vi "CRYStatistics Curve Op.vi"(0 "Data in":T1={"Name"="", "Curve"=[], "X data"=1, "Y data"=1, "Z data"=1, "X axis"=0, "Y axis"=1, "Z axis"=1, "X unit"="Hz", "Y unit"="", "Z unit"="deg.", "X dB ref"=1.0, "Y dB ref"=1.0, "Z dB ref"=1.0, "single val"=FALSE, "protected"=FALSE, "display X"=TRUE, "display Y"=TRUE, "display Z"=TRUE, "Test Info"="", "Step No."=0, "Plot Settings"={"Color"=0, "Interpolation"=0, "Point Style"=0, "Line Style"=0, "Point Color"=0, "Line Width"=0, "Bar Plot Style"=0, "Fill To"=0}, "AutoProtect"=FALSE} {"Z data" items=["dB", "Lin"]; "X data" items=["dB", "Lin"]; "Y data" items=["dB", "Lin"]; "Z dB ref" format="%.1f"; "Z axis" items=["Log", "Lin"]; "X dB ref" format="%.1f"; "X axis" items=["Log", "Lin"]; "Y axis" items=["Log", "Lin"]; "Y dB ref" format="%.1f"; "Curve"."z" format="%.2f"; "Curve"."y" format="%.2f"; "Curve"."x" format="%.2f"}, 1 "Sampling Rate":dbl, 2 "work in statics":u16, 4 "Statistical Operator":u16(ring) items=["Average", "Power Sum", "Maximum", "Minimum", "Est. Resonance", "Est. Notch", "IEEE TOLP", "IEEE ROLP", "IEEE SOLP", "ITU-T SLR", "ITU-T RLR", "ITU-T RLR w/Leak", "ITU-T STMR", "Attack Time", "Release Time", "Zwicker Loudness"], 5 "Wave":T4={"Waveform"={"X0"=0.0, "dX"=0.0, "Y"=[]}, "X data"=1, "Y data"=1, "Y axis"=1, "X unit"="s", "Y unit"="V", "Y dB ref"=1.0, "display Y"=TRUE, "display X"=TRUE, "Overload?"=FALSE, "Test Info"="", "Step No."=0, "Name"="", "protected"=FALSE, "Sqc history"=[], "Signal Channel ID"=0, "Plot Settings"={"Color"=0, "Interpolation"=0, "Point Style"=0, "Line Style"=0, "Point Color"=0, "Line Width"=0, "Bar Plot Style"=0, "Fill To"=0}, "AutoProtect"=FALSE} {"Y dB ref" format="%.1f"; "Y axis" items=["Log", "Lin"]; "Y data" items=["dB", "Lin"]; "X data" items=["dB", "Lin"]}, 7 "Search range":string[](array[string]), 8 "weight curve":string, 9 "All points":bool, 10 "Zwicker_spectrum":bool, 11 "Zwicker_X-axis":u16(ring) items=["Hz", "Bark"], 12 "Para_Resonance(%)":sgl format="%.2f", 13 "Use Default Value":bool, 14 "Curve/WFM ?":bool, 15 "Exponent":dbl) -> (17 "Q":dbl format="%.2f", 19 "Ranged data out(Curve)":T1={"Name"="", "Curve"=[], "X data"=1, "Y data"=1, "Z data"=1, "X axis"=0, "Y axis"=1, "Z axis"=1, "X unit"="Hz", "Y unit"="", "Z unit"="deg.", "X dB ref"=1.0, "Y dB ref"=1.0, "Z dB ref"=1.0, "single val"=FALSE, "protected"=FALSE, "display X"=TRUE, "display Y"=TRUE, "display Z"=TRUE, "Test Info"="", "Step No."=0, "Plot Settings"={"Color"=0, "Interpolation"=0, "Point Style"=0, "Line Style"=0, "Point Color"=0, "Line Width"=0, "Bar Plot Style"=0, "Fill To"=0}, "AutoProtect"=FALSE} {"Z data" items=["dB", "Lin"]; "X data" items=["dB", "Lin"]; "Y data" items=["dB", "Lin"]; "Z dB ref" format="%.1f"; "Z axis" items=["Log", "Lin"]; "X dB ref" format="%.1f"; "X axis" items=["Log", "Lin"]; "Y axis" items=["Log", "Lin"]; "Y dB ref" format="%.1f"; "Curve"."z" format="%.2f"; "Curve"."y" format="%.2f"; "Curve"."x" format="%.2f"}, 20 "Ranged data out(Value)":T1={"Name"="", "Curve"=[], "X data"=1, "Y data"=1, "Z data"=1, "X axis"=0, "Y axis"=1, "Z axis"=1, "X unit"="Hz", "Y unit"="", "Z unit"="deg.", "X dB ref"=1.0, "Y dB ref"=1.0, "Z dB ref"=1.0, "single val"=FALSE, "protected"=FALSE, "display X"=TRUE, "display Y"=TRUE, "display Z"=TRUE, "Test Info"="", "Step No."=0, "Plot Settings"={"Color"=0, "Interpolation"=0, "Point Style"=0, "Line Style"=0, "Point Color"=0, "Line Width"=0, "Bar Plot Style"=0, "Fill To"=0}, "AutoProtect"=FALSE} {"Z data" items=["dB", "Lin"]; "X data" items=["dB", "Lin"]; "Y data" items=["dB", "Lin"]; "Z dB ref" format="%.1f"; "Z axis" items=["Log", "Lin"]; "X dB ref" format="%.1f"; "X axis" items=["Log", "Lin"]; "Y axis" items=["Log", "Lin"]; "Y dB ref" format="%.1f"; "Curve"."z" format="%.2f"; "Curve"."y" format="%.2f"; "Curve"."x" format="%.2f"}, 21 "Frequency":dbl format="%.2f", 25 "index":i32, 27 "value":dbl format="%.2f")   [LabVIEW 2013]
uses:
  Typedef Control/CRYData Cluster.ctl
  Typedef Control/CRYWaveform Cluster.ctl
  Typedef Control/CRYCalibration 2DCluster.ctl
  Typedef Control/CRYCalibration Cluster.ctl
  <vilib>/Analysis/baseanly.llb/Mean (DBL).vi
  <vilib>/Analysis/NI_AALBase.lvlib
panel:
  in  "Calibration All Cluster":T2={"Calibration"={"Calibration Step Name"="", "Device"="", "Correction Curve Name"="", "Equalization Curve Name"="", "Sensitivity Curve Name"="", "Corr Folder and File"="", "EQ Folder and File"="", "Sens Folder and File"="", "Corr Step size"=0, "EQ Step size"=0, "Input"=FALSE, "Last Cal Date (sec)"=timestamp(0 s since 1904-01-01), "Cha Name"="", "Corr Curve Found"=FALSE, "EQ Curve Found"=FALSE, "Sens Curve Found"=FALSE, "Signal Type"="", "Calibrated Device"="", "Hz"=0}, "Corr Curve"={"Name"="", "Curve"=[], "X data"=1, "Y data"=1, "Z data"=1, "X axis"=0, "Y axis"=1, "Z axis"=1, "X unit"="Hz", "Y unit"="", "Z unit"="deg.", "X dB ref"=1.0, "Y dB ref"=1.0, "Z dB ref"=1.0, "single val"=FALSE, "protected"=FALSE, "display X"=TRUE, "display Y"=TRUE, "display Z"=TRUE, "Test Info"="", "Step No."=0, "Plot Settings"={"Color"=0, "Interpolation"=0, "Point Style"=0, "Line Style"=0, "Point Color"=0, "Line Width"=0, "Bar Plot Style"=0, "Fill To"=0}, "AutoProtect"=FALSE}, "EQ Curve"={"Name"="", "Curve"=[], "X data"=1, "Y data"=1, "Z data"=1, "X axis"=0, "Y axis"=1, "Z axis"=1, "X unit"="Hz", "Y unit"="", "Z unit"="deg.", "X dB ref"=1.0, "Y dB ref"=1.0, "Z dB ref"=1.0, "single val"=FALSE, "protected"=FALSE, "display X"=TRUE, "display Y"=TRUE, "display Z"=TRUE, "Test Info"="", "Step No."=0, "Plot Settings"={"Color"=0, "Interpolation"=0, "Point Style"=0, "Line Style"=0, "Point Color"=0, "Line Width"=0, "Bar Plot Style"=0, "Fill To"=0}, "AutoProtect"=FALSE}, "Sens Curve"={"Name"="", "Curve"=[], "X data"=1, "Y data"=1, "Z data"=1, "X axis"=0, "Y axis"=1, "Z axis"=1, "X unit"="Hz", "Y unit"="", "Z unit"="deg.", "X dB ref"=1.0, "Y dB ref"=1.0, "Z dB ref"=1.0, "single val"=FALSE, "protected"=FALSE, "display X"=TRUE, "display Y"=TRUE, "display Z"=TRUE, "Test Info"="", "Step No."=0, "Plot Settings"={"Color"=0, "Interpolation"=0, "Point Style"=0, "Line Style"=0, "Point Color"=0, "Line Width"=0, "Bar Plot Style"=0, "Fill To"=0}, "AutoProtect"=FALSE}} {"Sens Curve"."Z data" items=["dB", "Lin"]; "Sens Curve"."X data" items=["dB", "Lin"]; "Sens Curve"."Y data" items=["dB", "Lin"]; "Sens Curve"."Z dB ref" format="%.1f"; "Sens Curve"."Z axis" items=["Log", "Lin"]; "Sens Curve"."X dB ref" format="%.1f"; "Sens Curve"."X axis" items=["Log", "Lin"]; "Sens Curve"."Y axis" items=["Log", "Lin"]; "Sens Curve"."Y dB ref" format="%.1f"; "Sens Curve"."Curve"."z" format="%.2f"; "Sens Curve"."Curve"."y" format="%.2f"; "Sens Curve"."Curve"."x" format="%.2f"; "EQ Curve"."Z data" items=["dB", "Lin"]; "EQ Curve"."X data" items=["dB", "Lin"]; "EQ Curve"."Y data" items=["dB", "Lin"]; "EQ Curve"."Z dB ref" format="%.1f"; "EQ Curve"."Z axis" items=["Log", "Lin"]; "EQ Curve"."X dB ref" format="%.1f"; "EQ Curve"."X axis" items=["Log", "Lin"]; "EQ Curve"."Y axis" items=["Log", "Lin"]; "EQ Curve"."Y dB ref" format="%.1f"; "EQ Curve"."Curve"."z" format="%.2f"; "EQ Curve"."Curve"."y" format="%.2f"; "EQ Curve"."Curve"."x" format="%.2f"; "Corr Curve"."Z data" items=["dB", "Lin"]; "Corr Curve"."X data" items=["dB", "Lin"]; "Corr Curve"."Y data" items=["dB", "Lin"]; "Corr Curve"."Z dB ref" format="%.1f"; "Corr Curve"."Z axis" items=["Log", "Lin"]; "Corr Curve"."X dB ref" format="%.1f"; "Corr Curve"."X axis" items=["Log", "Lin"]; "Corr Curve"."Y axis" items=["Log", "Lin"]; "Corr Curve"."Y dB ref" format="%.1f"; "Corr Curve"."Curve"."z" format="%.2f"; "Corr Curve"."Curve"."y" format="%.2f"; "Corr Curve"."Curve"."x" format="%.2f"; "Calibration"."EQ Step size" items=["R10", "R20", "R40", "R80", "User"]; "Calibration"."Corr Step size" items=["R10", "R20", "R40", "R80", "User"]}
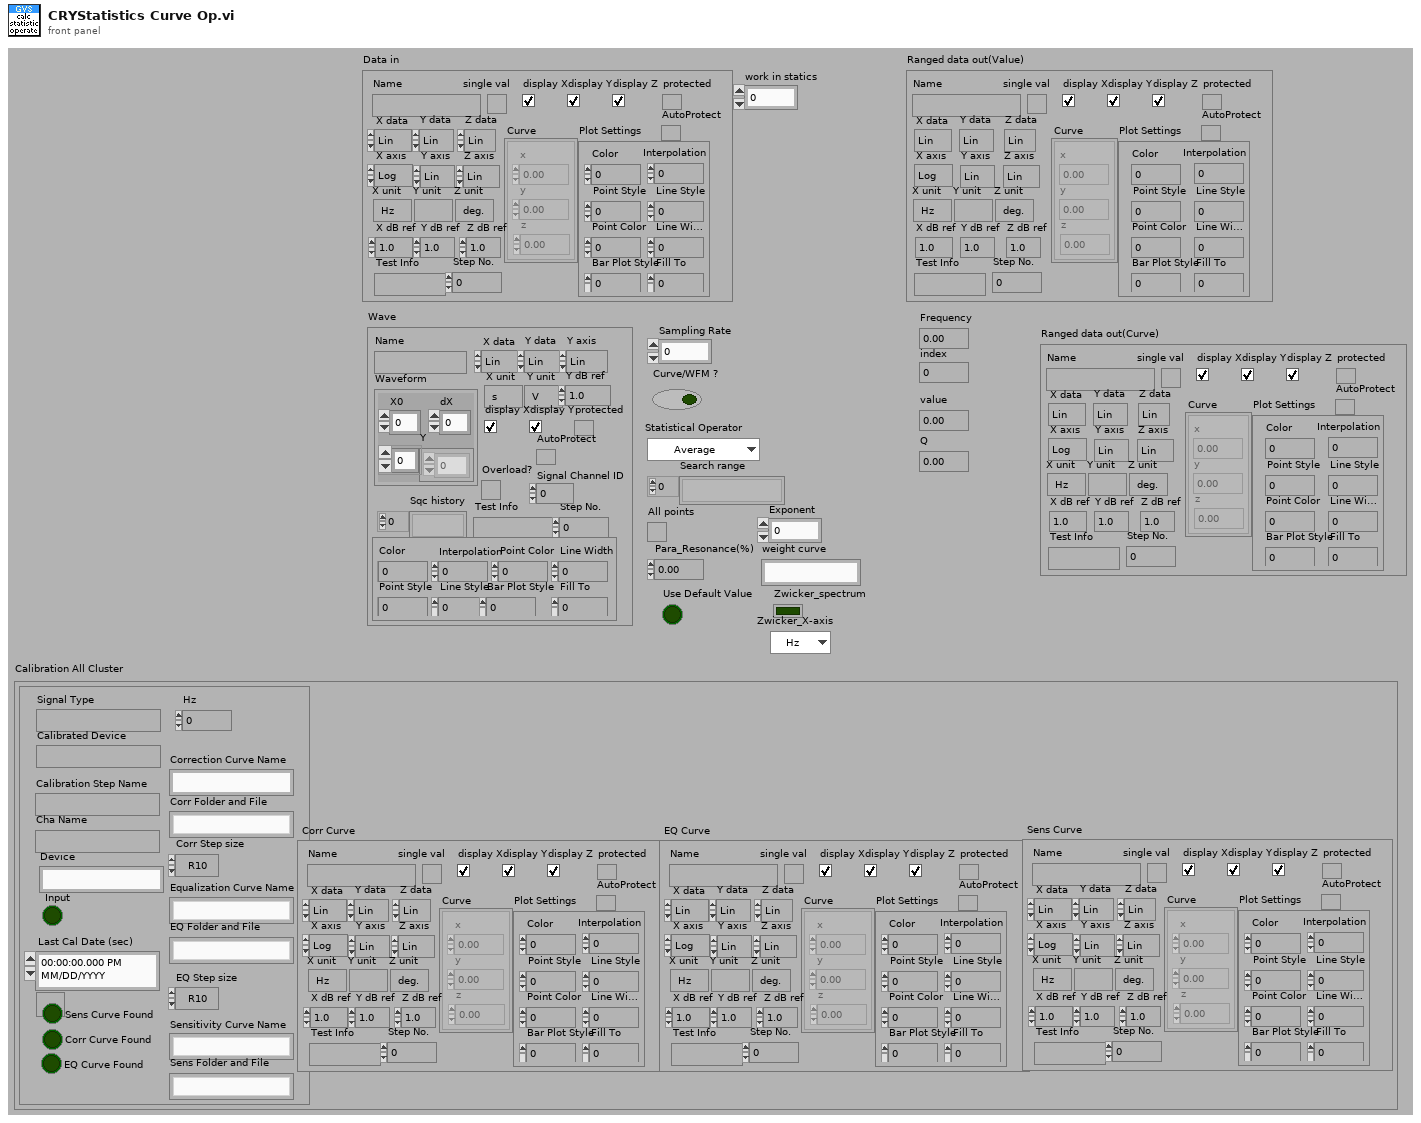
[diagram p1: front panel]
types:
  T1 = typedef "CRYData Cluster.ctl" = cluster{"Name":string, "Curve":cluster{"x":dbl, "y":dbl, "z":dbl}[], "X data":u16, "Y data":u16, "Z data":u16, "X axis":u16, "Y axis":u16, "Z axis":u16, "X unit":string, "Y unit":string, "Z unit":string, "X dB ref":dbl, "Y dB ref":dbl, "Z dB ref":dbl, "single val":bool, "protected":bool, "display X":bool, "display Y":bool, "display Z":bool, "Test Info":string, "Step No.":i32, "Plot Settings":cluster{"Color":u32, "Interpolation":u8, "Point Style":u8, "Line Style":u8, "Point Color":u32, "Line Width":u8, "Bar Plot Style":u8, "Fill To":i16}, "AutoProtect":bool}
  T2 = typedef "CRYCalibration 2DCluster.ctl" = cluster{"Calibration":T3, "Corr Curve":T1, "EQ Curve":T1, "Sens Curve":T1}
  T3 = typedef "CRYCalibration Cluster.ctl" = cluster{"Calibration Step Name":string, "Device":string, "Correction Curve Name":string, "Equalization Curve Name":string, "Sensitivity Curve Name":string, "Corr Folder and File":string, "EQ Folder and File":string, "Sens Folder and File":string, "Corr Step size":u16, "EQ Step size":u16, "Input":bool, "Last Cal Date (sec)":timestamp, "Cha Name":string, "Corr Curve Found":bool, "EQ Curve Found":bool, "Sens Curve Found":bool, "Signal Type":string, "Calibrated Device":string, "Hz":u32}
  T4 = typedef "CRYWaveform Cluster.ctl" = cluster{"Waveform":cluster{"X0":dbl, "dX":dbl, "Y":sgl[]}, "X data":u16, "Y data":u16, "Y axis":u16, "X unit":string, "Y unit":string, "Y dB ref":dbl, "display Y":bool, "display X":bool, "Overload?":bool, "Test Info":string, "Step No.":i32, "Name":string, "protected":bool, "Sqc history":string[], "Signal Channel ID":i32, "Plot Settings":cluster{"Color":u32, "Interpolation":u8, "Point Style":u8, "Line Style":u8, "Point Color":u32, "Line Width":u8, "Bar Plot Style":u8, "Fill To":i16}, "AutoProtect":bool}
  T5 = typedef "CRYStimulus Test Infor Cluster.ctl" = cluster{"Stimulus Type":string, "Signal Type":string, "In/Out":bool, "FAPS":cluster{"freq":dbl, "ampl":dbl, "cycles":dbl, "samples":i32}[], "Sampling Rate":dbl, "Samples":i32, "Analysis Param":string, "Resolution":u16, "Steps":u32, "Analysis Value":dbl[], "Diff Freq":dbl, "FStart":dbl, "FStop":dbl, "Calibration Param":string, "Anti Alias":dbl, "Level Out1":dbl, "Level Out2":dbl, "EQ":bool}
  T6 = cluster{"freq":dbl, "ampl":dbl, "cycles":dbl, "samples":i32}[]
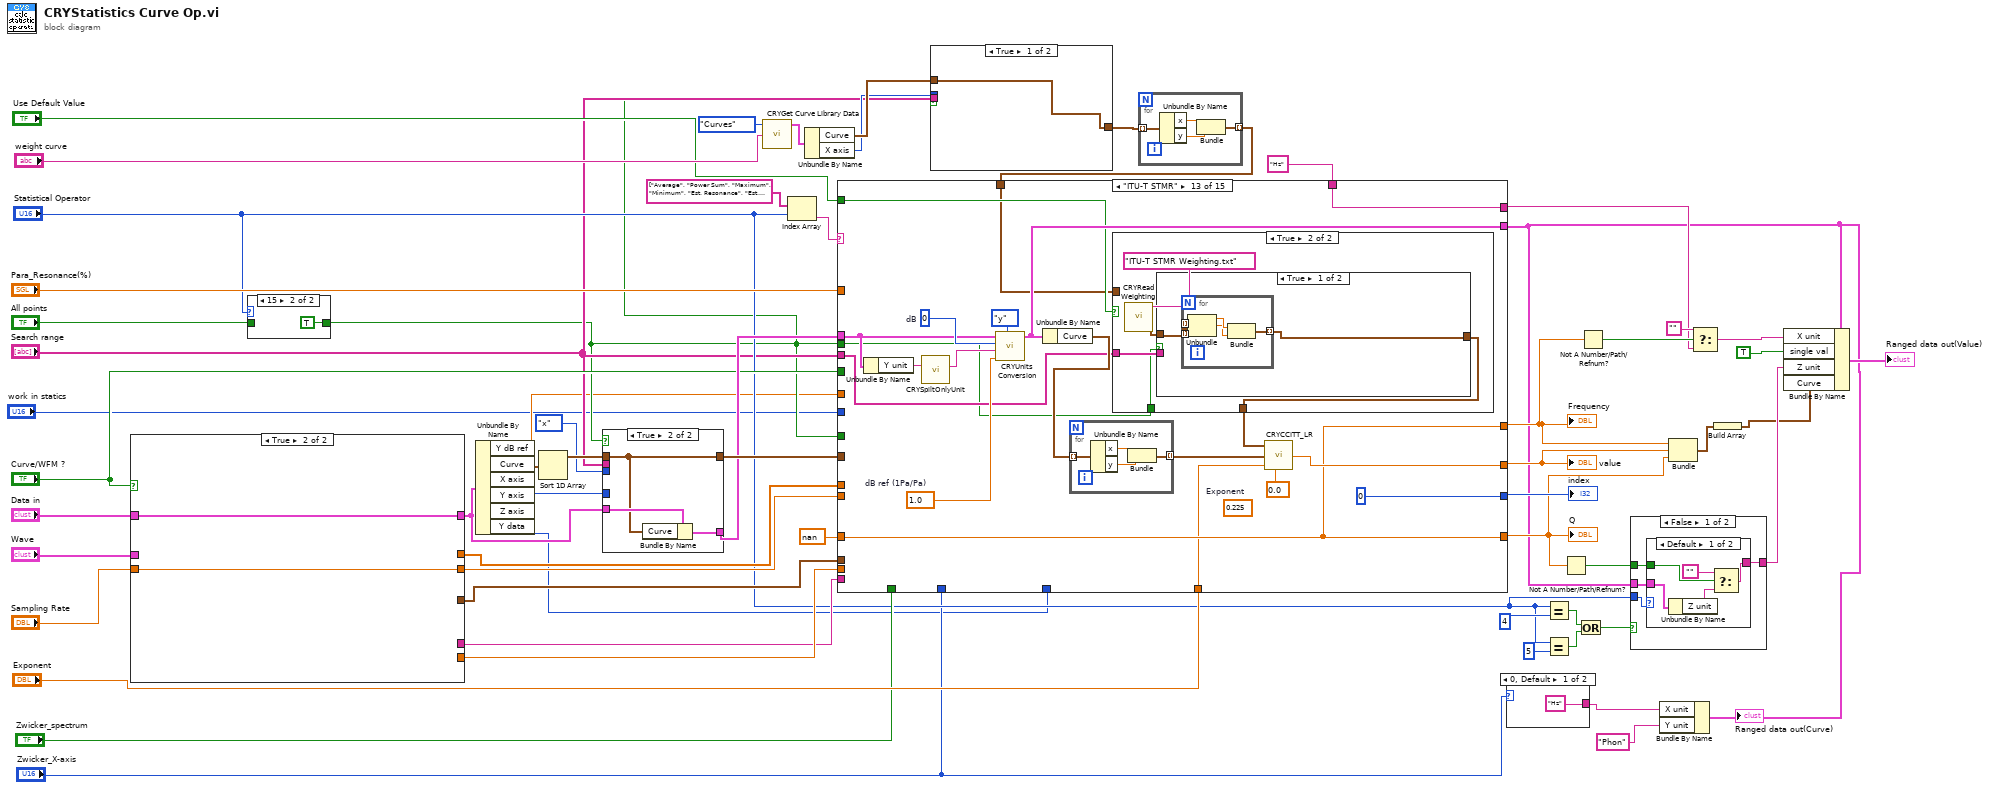
[diagram p0: block diagram]
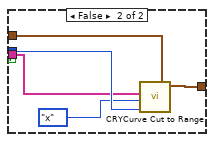
[diagram p2: hidden frame]
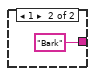
[diagram p3: hidden frame]
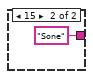
[diagram p5: hidden frame]
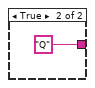
[diagram p6: hidden frame]
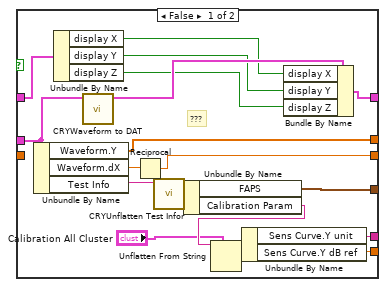
[diagram p7: hidden frame]
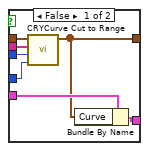
[diagram p8: hidden frame]
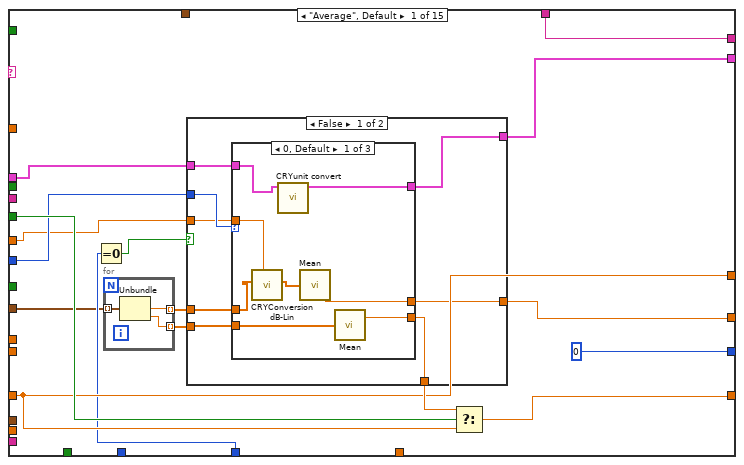
[diagram p9: hidden frame]
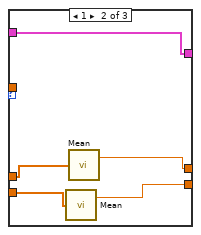
[diagram p10: hidden frame]
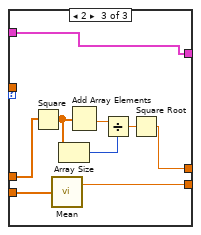
[diagram p11: hidden frame]
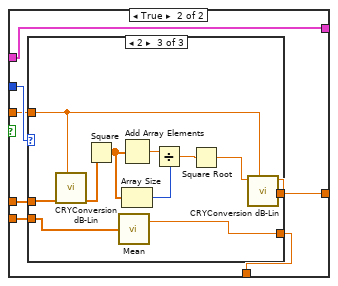
[diagram p12: hidden frame]
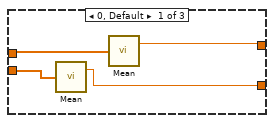
[diagram p13: hidden frame]
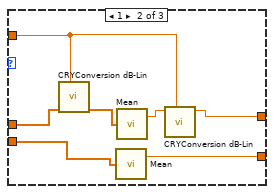
[diagram p14: hidden frame]
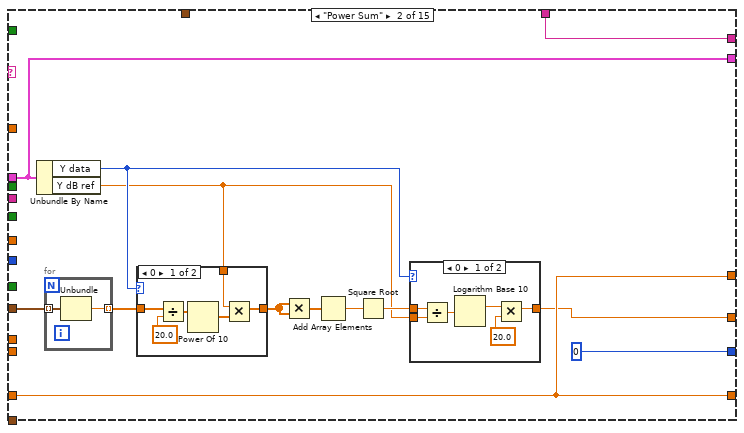
[diagram p15: hidden frame]
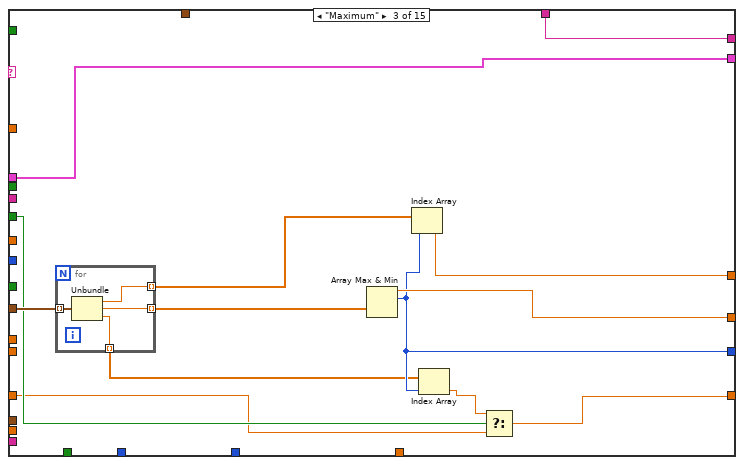
[diagram p18: hidden frame]
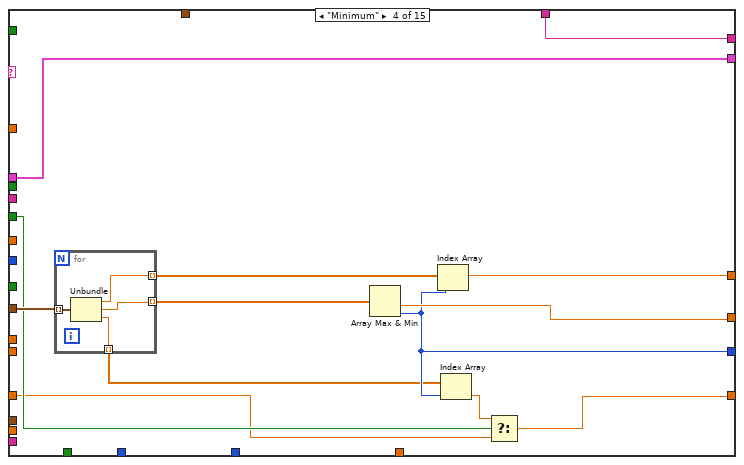
[diagram p19: hidden frame]
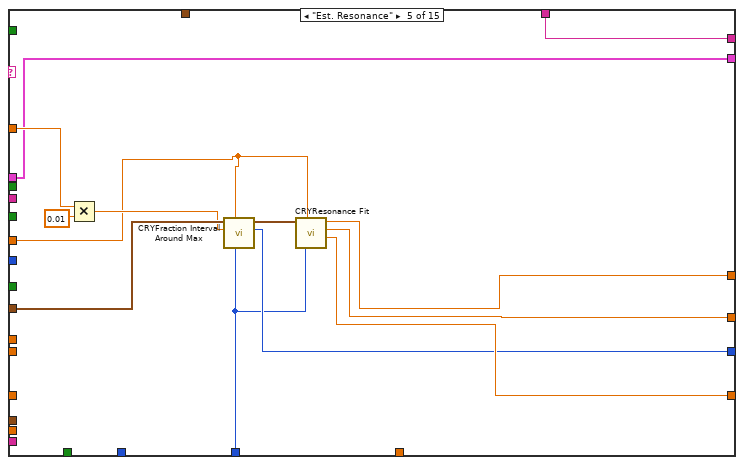
[diagram p20: hidden frame]
diagram:
  n1 = case shown="True" "Curve/WFM ?" {
    tunnel: "Data in" -> [w66 w82]
    tunnel: [w68 w82] -> w46
    tunnel: "Wave" -> [w80 _]
    tunnel: "Sampling Rate" -> [_ w81]
    tunnel: [w78 w81] -> w30
    tunnel: [w75 _] -> w29
    tunnel: [w74 _] -> w28
    tunnel: [w70 _] -> w27
    tunnel: [w69 _] -> w26
    frame False {
      # "???"
      n2 = Unbundle By Name(w80) -> ("Waveform.Y"=w74:sgl[], "Waveform.dX"=w79:dbl, "Test Info"=w77:string)
      n3 = Unbundle By Name(w66) -> ("display X"=w65:bool, "display Y"=w64:bool, "display Z"=w63:bool)
      n4 = call "CRYWaveform to DAT.vi"("Waveform In"=w80) -> ("Curve Out"=w67:T1)  [unwired: 10 out]
      n5 = Reciprocal(x=w79) -> (1/x=w78:dbl)
      n6 = call "CRYUnflatten Test Infor.vi"("Falattend test infor"=w77) -> ("unflattened test infor data"=w76:T5)  [unwired: 8 in, 1 out]
      n7 = Unbundle By Name(w76) -> ("FAPS"=w75:T6, "Calibration Param"=w73:string)
      n8 = Unflatten From String(type="Calibration All Cluster", binary string=w73) -> (value=w71:T2)  [unwired: 1 in, 4 out]
      n9 = Unbundle By Name(w71) -> ("Sens Curve.Y unit"=w69:string, "Sens Curve.Y dB ref"=w70:dbl)
      n10 = Bundle By Name(cluster=w67, "display X"=w65, "display Y"=w64, "display Z"=w63) -> (w68:T1)
    }
    frame True {
    }
  }
  n11 = case shown="15" "Statistical Operator" {
    tunnel: "All points" -> [w83 _]
    tunnel: [w83 TRUE ("All points")] -> w4
    frame Default {
    }
    frame 15 {
    }
  }
  n12 = Unbundle By Name(w46) -> ("Y dB ref"=w2:dbl, "Curve"=w60:cluster{"x":dbl, "y":dbl, "z":dbl}[], "X axis"=w55:u16, "Y data"=w3:u16)  [unwired: 2 out]
  n13 = Sort 1D Array(array=w60) -> (sorted array=w59:cluster{"x":dbl, "y":dbl, "z":dbl}[])
  n14 = case shown="True" w4 {
    tunnel: w59 -> [w91 w92]
    tunnel: [w87 w92] -> w53
    tunnel: enum16{"x", "y", "z"}."x" ("Range variable") -> [w90 _]
    tunnel: "Search range" -> [w89 _]
    tunnel: w46 -> [w88 w94]
    tunnel: [w86 w93] -> w44
    tunnel: w55 -> [w85 _]
    frame False {
      n15 = call "CRYCurve Cut to Range.vi"("Axis type (Lin)"=w85, "Range variable (x)"=w90, "Search range"=w89, "Curve in"=w91) -> ("Cut curve out"=w87:cluster{"x":dbl, "y":dbl, "z":dbl}[])  [unwired: 7 out]
      n16 = Bundle By Name(cluster=w88, "Curve"=w87) -> (w86:T1)
    }
    frame True {
      n17 = Bundle By Name(cluster=w94, "Curve"=w92) -> (w93:T1)
    }
  }
  n18 = call "CRYGet Curve Library Data.vi"("Type"=enum16{"Curves", "Values", "Results", "WFM"}."Curves", "Data Name"="weight curve") -> ("Curve"=w19:T1)  [unwired: 4 out]
  n19 = Index Array(array=string[] ["Average", "Power Sum", "Maximum", "Minimum", "Est. Resonance", "Est. Notch", "IEEE TOLR", "IEEE ROLR", "IEEE SOLR", "ITU-T SLR", "ITU-T RLR", "ITU-T RLR w/ Leak", "ITU-T STMR", "Attack Time", "Release Time", "Zwicker Loudness"] ("Scalar Op Name"), index="Statistical Operator") -> (element=w54:string)
  n20 = Unbundle By Name(w19) -> ("Curve"=w9:cluster{"x":dbl, "y":dbl, "z":dbl}[], "X axis"=w7:u16)
  n21 = case shown="True" w4 {
    tunnel: w9 -> [w95 w100]
    tunnel: [w95 w99] -> w8
    tunnel: w7 -> [_ w98]
    tunnel: "Search range" -> [_ w97]
    frame True {
    }
    frame False {
      n22 = call "CRYCurve Cut to Range.vi"("Axis type (Lin)"=w98, "Range variable (x)"=enum16{"x", "y", "z"}."x" ("Range variable"), "Search range"=w97, "Curve in"=w100) -> ("Cut curve out"=w99:cluster{"x":dbl, "y":dbl, "z":dbl}[])  [unwired: 7 out]
    }
  }
  n23 = for {
    tunnel: w8 -> [w104] mode=indexing
    tunnel: [w101] -> w5 mode=indexing
    n24 = Unbundle By Name(w104) -> ("x"=w103:dbl, "y"=w102:dbl)
    n25 = Bundle("x"=w103, "y"=w102) -> (w101:cluster{"x":dbl, "y":dbl})  [unwired: 1 out]
  }
  n26 = case shown="\"ITU-T STMR\"" w54 {
    selector: w54 -> [_ _ _ _ _ _ _ _ _ _ _ _ _ w515 _]
    tunnel: w53 -> [w111 w195 w224 w241 w253 w265 _ _ _ _ _ _ _ _ _]
    tunnel: [w120 w186 w223 w240 w250 w263 w285 w304 w323 w343 w390 w436 w482 w513 w548] -> w40
    tunnel: [w115 w193 w222 w239 w251 w264 w279 w298 w317 w340 w386 w432 w478 w518 w549] -> w41
    tunnel: [0 0 w218 w235 w248 w266 0 0 0 0 0 0 0 0 _] -> w52
    tunnel: w44 -> [w106 w184 w219 w236 w256 w271 w274 w292 w311 w335 w381 w427 w473 w538 w546]
    tunnel: [w105 w184 w219 w236 w256 w271 w277 w296 w315 w339 w385 w431 w477 w537 w544] -> w14
    tunnel: [w114 w193 w212 w229 w249 w262 w279 w298 w317 w340 w386 w432 w478 w532 w547] -> w39
    tunnel: nan -> [w115 w193 w213 w230 _ _ w279 w298 w317 w340 w386 w432 w478 w532 _]
    tunnel: "Para_Resonance(%)" -> [_ _ _ _ w258 w269 _ _ _ _ _ _ _ w540 _]
    tunnel: w30 -> [_ _ _ _ _ _ _ _ _ _ _ _ _ w542 _]
    tunnel: "Search range" -> [_ _ _ _ _ _ _ _ _ w331 w376 w422 w468 w536 _]
    tunnel: w4 -> [_ _ _ _ _ _ _ _ _ _ w375 w421 w467 w535 _]
    tunnel: w29 -> [_ _ _ _ _ _ _ _ _ _ _ _ _ w534 _]
    tunnel: w28 -> [_ _ _ _ _ _ _ _ _ _ _ _ _ w533 _]
    tunnel: w27 -> [_ _ _ _ _ _ _ _ _ _ _ _ _ w519 _]
    tunnel: w26 -> [_ _ _ _ _ _ _ _ _ _ _ _ _ w524 _]
    tunnel: "Hz" -> [w118 w183 w216 w233 w255 w268 w276 w295 w314 w338 w384 w430 w476 _ _]
    tunnel: [w118 w183 w216 w233 w255 w268 w276 w295 w314 w338 w384 w430 w476 "s" "Phon"] -> w24
    tunnel: "Curve/WFM ?" -> [w117 _ w215 w232 _ _ _ _ _ _ _ _ _ _ _]
    tunnel: "Exponent" -> [_ _ _ _ _ _ w275 w294 w313 w337 w383 w429 w475 _ _]
    tunnel: w5 -> [_ _ _ _ _ _ _ _ _ w332 w377 w423 w470 _ _]
    tunnel: "Use Default Value" -> [_ _ _ _ _ _ _ _ _ w333 w379 w424 w471 _ _]
    tunnel: "Zwicker_spectrum" -> [_ _ _ _ _ _ _ _ _ _ _ _ _ _ w550]
    tunnel: "Zwicker_X-axis" -> [_ _ _ _ _ _ _ _ _ _ _ _ _ _ w551]
    tunnel: w4 -> [_ _ _ _ _ _ _ _ _ w330 _ _ _ _ _]
    tunnel: w3 -> [w113 _ _ _ w247 w259 _ _ _ _ _ _ _ _ _]
    tunnel: w2 -> [w107 _ _ _ w246 w261 _ _ _ _ _ _ _ _ _]
    tunnel: "work in statics" -> [w108 _ _ _ _ _ _ _ _ _ _ _ _ _ _]
    frame "Average", Default {
      n27 = Equal To 0?(x=w113) -> (x = 0?=w112:bool)
      n28 = for {
        tunnel: w111 -> [w123] mode=indexing
        tunnel: [w122] -> w110 mode=indexing
        tunnel: [w121] -> w109 mode=indexing
        n29 = Unbundle(w123) -> ("y"=w122:dbl, "z"=w121:dbl)  [unwired: 1 out]
      }
      n30 = case shown="False" w112 {
        tunnel: [w128 w160] -> w120
        tunnel: [w129 w159] -> w116
        tunnel: w110 -> [w131 w158]
        tunnel: w109 -> [w130 w157]
        tunnel: w108 -> [w127 w156]
        tunnel: w107 -> [w126 w155]
        tunnel: w106 -> [w125 w154]
        tunnel: [w124 w154] -> w105
        frame False {
          n31 = case shown="0, Default" w127 {
            tunnel: w131 -> [w137 w144 w150]
            tunnel: w130 -> [w139 w142 w149]
            tunnel: [w138 w141 w148] -> w129
            tunnel: [w135 w143 w146] -> w128
            tunnel: w126 -> [w134 _ _]
            tunnel: w125 -> [w133 w140 w145]
            tunnel: [w132 w140 w145] -> w124
            frame 0, Default {
              n32 = call "CRYConversion dB-Lin.vi"("dB ref."=w134, "Lin In array"=w137) -> ("Log Out array"=w136:dbl[])  [unwired: 4 in, 3 out]
              n33 = call "CRYunit convert.vi"("A data for units"=w133) -> ("Result out"=w132:T1)  [unwired: 10 in]
              n34 = call-poly <vilib>:"Mean.vi"("X"=w136) -> ("mean"=w135:dbl)  [unwired: 1 out]
              n35 = call-poly <vilib>:"Mean.vi"("X"=w139) -> ("mean"=w138:dbl)  [unwired: 1 out]
            }
            frame 1 {
              n36 = call-poly <vilib>:"Mean.vi"("X"=w142) -> ("mean"=w141:dbl)  [unwired: 1 out]
              n37 = call-poly <vilib>:"Mean.vi"("X"=w144) -> ("mean"=w143:dbl)  [unwired: 1 out]
            }
            frame 2 {
              n38 = Square(x=w150) -> (x^2=w152:dbl[])
              n39 = call-poly <vilib>:"Mean.vi"("X"=w149) -> ("mean"=w148:dbl)  [unwired: 1 out]
              n40 = Array Size(array=w152) -> (size(s)=w151:i32)
              n41 = Add Array Elements(numeric array=w152) -> (sum=w153:dbl)
              n42 = Divide(x=w153, y=w151) -> (x/y=w147:dbl)
              n43 = Square Root(x=w147) -> (sqrt(x)=w146:dbl)
            }
          }
        }
        frame True {
          n44 = case shown="2" w156 {
            tunnel: [w161 w166 w175] -> w160
            tunnel: [w163 w171 w176] -> w159
            tunnel: w158 -> [w162 w169 w182]
            tunnel: w157 -> [w164 w170 w177]
            tunnel: w155 -> [_ w165 w174]
            frame 0, Default {
              n45 = call-poly <vilib>:"Mean.vi"("X"=w164) -> ("mean"=w163:dbl)  [unwired: 1 out]
              n46 = call-poly <vilib>:"Mean.vi"("X"=w162) -> ("mean"=w161:dbl)  [unwired: 1 out]
            }
            frame 1 {
              n47 = call "CRYConversion dB-Lin.vi"("dB ref."=w165, "Log In array"=w169) -> ("Lin Out array"=w168:dbl[])  [unwired: 4 in, 3 out]
              n48 = call-poly <vilib>:"Mean.vi"("X"=w170) -> ("mean"=w171:dbl)  [unwired: 1 out]
              n49 = call-poly <vilib>:"Mean.vi"("X"=w168) -> ("mean"=w167:dbl)  [unwired: 1 out]
              n50 = call "CRYConversion dB-Lin.vi"("dB ref."=w165, "Lin In"=w167) -> ("Log Out"=w166:dbl)  [unwired: 4 in, 3 out]
            }
            frame 2 {
              n51 = call "CRYConversion dB-Lin.vi"("dB ref."=w174, "Log In array"=w182) -> ("Lin Out array"=w178:dbl[])  [unwired: 4 in, 3 out]
              n52 = Square(x=w178) -> (x^2=w180:dbl[])
              n53 = call-poly <vilib>:"Mean.vi"("X"=w177) -> ("mean"=w176:dbl)  [unwired: 1 out]
              n54 = Add Array Elements(numeric array=w180) -> (sum=w181:dbl)
              n55 = Array Size(array=w180) -> (size(s)=w179:i32)
              n56 = Divide(x=w181, y=w179) -> (x/y=w173:dbl)
              n57 = Square Root(x=w173) -> (sqrt(x)=w172:dbl)
              n58 = call "CRYConversion dB-Lin.vi"("dB ref."=w174, "Lin In"=w172) -> ("Log Out"=w175:dbl)  [unwired: 4 in, 3 out]
            }
          }
        }
      }
      n59 = Select(t=w116, s=w117, f=w115) -> (s? t:f=w114:dbl)
    }
    frame "Power Sum" {
      n60 = Unbundle By Name(w184) -> ("Y data"=w191:u16, "Y dB ref"=w185:dbl)
      n61 = for {
        tunnel: w195 -> [w211] mode=indexing
        tunnel: [w210] -> w192 mode=indexing
        n62 = Unbundle(w211) -> ("y"=w210:dbl)  [unwired: 2 out]
      }
      n63 = case shown="0" w191 {
        tunnel: [w203 w209] -> w190
        tunnel: w192 -> [w208 w209]
        tunnel: w185 -> [w204 _]
        frame 0 {
          n64 = Divide(x=w208, y=20.0) -> (x/y=w206:dbl[])
          n65 = Power Of 10(x=w206) -> (10^x=w205:dbl[])
          n66 = Multiply(x=w204, y=w205) -> (x*y=w203:dbl[])
        }
        frame 1, Default {
        }
      }
      n67 = Multiply(x=w190, y=w190) -> (x*y=w189:dbl[])
      n68 = Add Array Elements(numeric array=w189) -> (sum=w188:dbl)
      n69 = Square Root(x=w188) -> (sqrt(x)=w187:dbl)
      n70 = case shown="0" w191 {
        tunnel: w187 -> [w201 w202]
        tunnel: [w196 w202] -> w186
        tunnel: w185 -> [w200 _]
        frame 0 {
          n71 = Divide(x=w201, y=w200) -> (x/y=w199:dbl)
          n72 = Logarithm Base 10(1:w199) -> (0:w198:dbl)
          n73 = Multiply(x=w198, y=20.0 ("x")) -> (x*y=w196:dbl)
        }
        frame 1, Default {
        }
      }
    }
    frame "Maximum" {
      n74 = for {
        tunnel: w224 -> [w228] mode=indexing
        tunnel: [w226] -> w221 mode=indexing
        tunnel: [w227] -> w220 mode=indexing
        tunnel: [w225] -> w217 mode=indexing
        n75 = Unbundle(w228) -> ("x"=w226:dbl, "y"=w227:dbl, "z"=w225:dbl)
      }
      n76 = Array Max & Min(array=w220) -> (max value=w223:dbl, max index (indices)=w218:i32)  [unwired: 2 out]
      n77 = Index Array(array=w221, index=w218) -> (element=w222:dbl)
      n78 = Index Array(array=w217, index=w218) -> (element=w214:dbl)
      n79 = Select(t=w214, s=w215, f=w213) -> (s? t:f=w212:dbl)
    }
    frame "Minimum" {
      n80 = for {
        tunnel: w241 -> [w245] mode=indexing
        tunnel: [w244] -> w238 mode=indexing
        tunnel: [w243] -> w237 mode=indexing
        tunnel: [w242] -> w234 mode=indexing
        n81 = Unbundle(w245) -> ("x"=w243:dbl, "y"=w244:dbl, "z"=w242:dbl)
      }
      n82 = Array Max & Min(array=w238) -> (min value=w240:dbl, min index (indices)=w235:i32)  [unwired: 2 out]
      n83 = Index Array(array=w237, index=w235) -> (element=w239:dbl)
      n84 = Index Array(array=w234, index=w235) -> (element=w231:dbl)
      n85 = Select(t=w231, s=w232, f=w230) -> (s? t:f=w229:dbl)
    }
    frame "Est. Resonance" {
      n86 = Multiply(x=w258, y=0.01) -> (x*y=w252:dbl)
      n87 = call "CRYFraction Interval Around Max.vi"("Y data"=w247, "Y ref"=w246, "Fraction down (1/sqrt(2))"=w252, "Curve in"=w253) -> ("Index"=w248:i32, "Interval around max"=w254:cluster{"Freq":dbl, "Magn":dbl}[])  [unwired: 6 out]
      n88 = call "CRYResonance Fit.vi"("Y data"=w247, "Y ref"=w246, "Input"=w254) -> ("Q"=w249:dbl, "Magn"=w250:dbl, "Freq"=w251:dbl)  [unwired: 1 in, 5 out]
    }
    frame "Est. Notch" {
      n89 = Multiply(x=w269, y=0.01) -> (x*y=w267:dbl)
      n90 = call "CRYNot.ch Resonance.vi"("Y ref"=w261, "Curve in"=w265, "Fraction down (1/sqrt(2))"=w267, "Y data"=w259) -> ("Index"=w266:i32, "Interval around max"=w260:cluster{"Freq":dbl, "Magn":dbl}[])  [unwired: 6 in]
      n91 = call "CRYNotch Resonance Results.vi"("Y ref"=w261, "Input"=w260, "Y data"=w259) -> ("Q"=w262:dbl, "Magn"=w263:dbl, "Freq"=w264:dbl)  [unwired: 5 in, 1 out]
    }
    frame "IEEE TOLR" {
      w278 = 0.0  # dB Correction [dB]
      w280 = u16 0  # dB
      w281 = 0.001  # dB ref (1mV/Pa)
      n92 = Unbundle By Name(w274) -> ("Y unit"=w273:string)
      n93 = call "CRYSpiltOnlyUnit.vi"("In Unit String"=w273) -> ("Out Unit String"=w272:string)  [unwired: 10 in]
      n94 = call "CRYUnits Conversion.vi"("Axis to change units"=enum16{"x", "y", "z"}."y", "New dB ref"=w281, "Custom unit in"=w272, "New data (dB/Lin)"=w280, "Data in"=w274) -> ("Data with new units"=w277:T1)  [unwired: 6 out]
      n95 = Unbundle By Name(w277) -> ("Curve"=w282:cluster{"x":dbl, "y":dbl, "z":dbl}[])
      n96 = for {
        tunnel: w282 -> [w290] mode=indexing
        tunnel: [w287] -> w286 mode=indexing
        n97 = Unbundle By Name(w290) -> ("x"=w289:dbl, "y"=w288:dbl)
        n98 = Bundle("x"=w289, "y"=w288) -> (w287:cluster{"x":dbl, "y":dbl})  [unwired: 1 out]
      }
      n99 = call "CRYOLR.vi"("Freq. Response [Hz,dB]"=w286, "Exponent"=w275, "dB Correction [dB]"=w278) -> ("OLR [dB]"=w285:dbl)  [unwired: 2 in]
    }
    frame "IEEE ROLR" {
      w297 = 0.0  # dB Correction [dB]
      w299 = u16 0  # dB
      w300 = 1000.0  # dB ref (1Pa/mV)
      n100 = Unbundle By Name(w292) -> ("Y unit"=w293:string)
      n101 = call "CRYSpiltOnlyUnit.vi"("In Unit String"=w293) -> ("Out Unit String"=w291:string)  [unwired: 10 in]
      n102 = call "CRYUnits Conversion.vi"("Axis to change units"=enum16{"x", "y", "z"}."y", "New dB ref"=w300, "Custom unit in"=w291, "New data (dB/Lin)"=w299, "Data in"=w292) -> ("Data with new units"=w296:T1)  [unwired: 6 out]
      n103 = Unbundle By Name(w296) -> ("Curve"=w301:cluster{"x":dbl, "y":dbl, "z":dbl}[])
      n104 = for {
        tunnel: w301 -> [w309] mode=indexing
        tunnel: [w306] -> w305 mode=indexing
        n105 = Unbundle By Name(w309) -> ("x"=w308:dbl, "y"=w307:dbl)
        n106 = Bundle("x"=w308, "y"=w307) -> (w306:cluster{"x":dbl, "y":dbl})  [unwired: 1 out]
      }
      n107 = call "CRYOLR.vi"("Freq. Response [Hz,dB]"=w305, "Exponent"=w294, "dB Correction [dB]"=w297) -> ("OLR [dB]"=w304:dbl)  [unwired: 2 in]
    }
    frame "IEEE SOLR" {
      w316 = 0.0  # dB Correction [dB]
      w318 = u16 0  # dB
      w319 = 1.0  # dB ref (1Pa/Pa)
      n108 = Unbundle By Name(w311) -> ("Y unit"=w312:string)
      n109 = call "CRYSpiltOnlyUnit.vi"("In Unit String"=w312) -> ("Out Unit String"=w310:string)  [unwired: 10 in]
      n110 = call "CRYUnits Conversion.vi"("Axis to change units"=enum16{"x", "y", "z"}."y", "New dB ref"=w319, "Custom unit in"=w310, "New data (dB/Lin)"=w318, "Data in"=w311) -> ("Data with new units"=w315:T1)  [unwired: 6 out]
      n111 = Unbundle By Name(w315) -> ("Curve"=w320:cluster{"x":dbl, "y":dbl, "z":dbl}[])
      n112 = for {
        tunnel: w320 -> [w328] mode=indexing
        tunnel: [w325] -> w324 mode=indexing
        n113 = Unbundle By Name(w328) -> ("x"=w327:dbl, "y"=w326:dbl)
        n114 = Bundle("x"=w327, "y"=w326) -> (w325:cluster{"x":dbl, "y":dbl})  [unwired: 1 out]
      }
      n115 = call "CRYOLR.vi"("Freq. Response [Hz,dB]"=w324, "Exponent"=w313, "dB Correction [dB]"=w316) -> ("OLR [dB]"=w323:dbl)  [unwired: 2 in]
    }
    frame "ITU-T SLR" {
      w342 = u16 0  # dB
      (unwired) 0.175  # Exponent
      w346 = 1.0  # dB ref (1V/Pa)
      n116 = Unbundle By Name(w335) -> ("Y unit"=w336:string)
      n117 = call "CRYSpiltOnlyUnit.vi"("In Unit String"=w336) -> ("Out Unit String"=w334:string)  [unwired: 10 in]
      n118 = call "CRYUnits Conversion.vi"("Axis to change units"=enum16{"x", "y", "z"}."y", "New dB ref"=w346, "Custom unit in"=w334, "New data (dB/Lin)"=w342, "Data in"=w335) -> ("Data with new units"=w339:T1)  [unwired: 6 out]
      n119 = Unbundle By Name(w339) -> ("Curve"=w345:cluster{"x":dbl, "y":dbl, "z":dbl}[])
      n120 = for {
        tunnel: w345 -> [w374] mode=indexing
        tunnel: [w371] -> w344 mode=indexing
        n121 = Unbundle By Name(w374) -> ("x"=w373:dbl, "y"=w372:dbl)
        n122 = Bundle("x"=w373, "y"=w372) -> (w371:cluster{"x":dbl, "y":dbl})  [unwired: 1 out]
      }
      n123 = case shown="True" w333 {
        tunnel: [w349 w350] -> w329
        tunnel: w332 -> [w349 _]
        tunnel: w331 -> [_ w352]
        tunnel: w330 -> [_ w351]
        frame False {
        }
        frame True {
          n124 = call "CRYRead Weighting.vi"("Weighting filename"="ITU-T SLR Weighting.txt") -> ("Array"=w353:cluster{dbl, dbl, dbl}[])  [unwired: 9 in]
          n125 = case shown="False" w351 {
            tunnel: w353 -> [w356 w366]
            tunnel: w352 -> [_ w364]
            tunnel: [w355 w361] -> w350
            frame True {
              n126 = for {
                tunnel: [w360] -> w355 mode=indexing
                tunnel: w356 -> [w359] mode=indexing
                n127 = Unbundle(w359) -> (w358:dbl, w357:dbl)  [unwired: 1 out]
                n128 = Bundle(w358, w357) -> (w360:cluster{dbl, dbl})  [unwired: 1 out]
              }
            }
            frame False {
              n129 = call "CRYCurve Cut to Range.vi"("Axis type (Lin)"=0, "Range variable (x)"=enum16{"x", "y", "z"}."x" ("Range variable"), "Search range"=w364, "Curve in"=w366) -> ("Cut curve out"=w362:cluster{"x":dbl, "y":dbl, "z":dbl}[])  [unwired: 7 out]
              n130 = for {
                tunnel: w362 -> [w370] mode=indexing
                tunnel: [w367] -> w361 mode=indexing
                n131 = Unbundle By Name(w370) -> ("x"=w369:dbl, "y"=w368:dbl)
                n132 = Bundle("x"=w369, "y"=w368) -> (w367:cluster{"x":dbl, "y":dbl})  [unwired: 1 out]
              }
            }
          }
        }
      }
      n133 = call "CRYCCITT_LR.vi"("Weight [Hz,dB]"=w329, "Freq. Response [Hz,dB]"=w344, "Exponent"=w337, "dB Correction [dB]"=0.0) -> ("LR [dB]"=w343:dbl)  [unwired: 1 out]
    }
    frame "ITU-T RLR" {
      w388 = u16 0  # dB
      w389 = 1.0  # dB ref (1Pa/V)
      (unwired) 0.175  # Exponent
      n134 = Unbundle By Name(w381) -> ("Y unit"=w382:string)
      n135 = call "CRYSpiltOnlyUnit.vi"("In Unit String"=w382) -> ("Out Unit String"=w380:string)  [unwired: 10 in]
      n136 = call "CRYUnits Conversion.vi"("Axis to change units"=enum16{"x", "y", "z"}."y", "New dB ref"=w389, "Custom unit in"=w380, "New data (dB/Lin)"=w388, "Data in"=w381) -> ("Data with new units"=w385:T1)  [unwired: 6 out]
      n137 = Unbundle By Name(w385) -> ("Curve"=w392:cluster{"x":dbl, "y":dbl, "z":dbl}[])
      n138 = for {
        tunnel: w392 -> [w420] mode=indexing
        tunnel: [w417] -> w391 mode=indexing
        n139 = Unbundle By Name(w420) -> ("x"=w419:dbl, "y"=w418:dbl)
        n140 = Bundle("x"=w419, "y"=w418) -> (w417:cluster{"x":dbl, "y":dbl})  [unwired: 1 out]
      }
      n141 = case shown="True" w379 {
        tunnel: [w395 w396] -> w378
        tunnel: w377 -> [w395 _]
        tunnel: w376 -> [_ w398]
        tunnel: w375 -> [_ w397]
        frame False {
        }
        frame True {
          n142 = call "CRYRead Weighting.vi"("Weighting filename"="ITU-T RLR Weighting.txt") -> ("Array"=w399:cluster{dbl, dbl, dbl}[])  [unwired: 9 in]
          n143 = case shown="False" w397 {
            tunnel: w399 -> [w402 w412]
            tunnel: w398 -> [_ w410]
            tunnel: [w401 w407] -> w396
            frame True {
              n144 = for {
                tunnel: [w406] -> w401 mode=indexing
                tunnel: w402 -> [w405] mode=indexing
                n145 = Unbundle(w405) -> (w404:dbl, w403:dbl)  [unwired: 1 out]
                n146 = Bundle(w404, w403) -> (w406:cluster{dbl, dbl})  [unwired: 1 out]
              }
            }
            frame False {
              n147 = call "CRYCurve Cut to Range.vi"("Axis type (Lin)"=0, "Range variable (x)"=enum16{"x", "y", "z"}."x" ("Range variable"), "Search range"=w410, "Curve in"=w412) -> ("Cut curve out"=w408:cluster{"x":dbl, "y":dbl, "z":dbl}[])  [unwired: 7 out]
              n148 = for {
                tunnel: w408 -> [w416] mode=indexing
                tunnel: [w413] -> w407 mode=indexing
                n149 = Unbundle By Name(w416) -> ("x"=w415:dbl, "y"=w414:dbl)
                n150 = Bundle("x"=w415, "y"=w414) -> (w413:cluster{"x":dbl, "y":dbl})  [unwired: 1 out]
              }
            }
          }
        }
      }
      n151 = call "CRYCCITT_LR.vi"("Weight [Hz,dB]"=w378, "Freq. Response [Hz,dB]"=w391, "Exponent"=w383, "dB Correction [dB]"=0.0) -> ("LR [dB]"=w390:dbl)  [unwired: 1 out]
    }
    frame "ITU-T RLR w/ Leak" {
      w434 = u16 0  # dB
      w435 = 1.0  # dB ref (1Pa/V)
      (unwired) 0.175  # Exponent
      n152 = Unbundle By Name(w427) -> ("Y unit"=w428:string)
      n153 = call "CRYSpiltOnlyUnit.vi"("In Unit String"=w428) -> ("Out Unit String"=w426:string)  [unwired: 10 in]
      n154 = call "CRYUnits Conversion.vi"("Axis to change units"=enum16{"x", "y", "z"}."y", "New dB ref"=w435, "Custom unit in"=w426, "New data (dB/Lin)"=w434, "Data in"=w427) -> ("Data with new units"=w431:T1)  [unwired: 6 out]
      n155 = Unbundle By Name(w431) -> ("Curve"=w438:cluster{"x":dbl, "y":dbl, "z":dbl}[])
      n156 = for {
        tunnel: w438 -> [w466] mode=indexing
        tunnel: [w463] -> w437 mode=indexing
        n157 = Unbundle By Name(w466) -> ("x"=w465:dbl, "y"=w464:dbl)
        n158 = Bundle("x"=w465, "y"=w464) -> (w463:cluster{"x":dbl, "y":dbl})  [unwired: 1 out]
      }
      n159 = case shown="True" w424 {
        tunnel: [w441 w442] -> w425
        tunnel: w423 -> [w441 _]
        tunnel: w422 -> [_ w444]
        tunnel: w421 -> [_ w443]
        frame False {
        }
        frame True {
          n160 = call "CRYRead Weighting.vi"("Weighting filename"="ITU-T RLR with Leakage Weighting.txt") -> ("Array"=w445:cluster{dbl, dbl, dbl}[])  [unwired: 9 in]
          n161 = case shown="True" w443 {
            tunnel: w445 -> [w448 w458]
            tunnel: w444 -> [_ w457]
            tunnel: [w447 w453] -> w442
            frame True {
              n162 = for {
                tunnel: [w452] -> w447 mode=indexing
                tunnel: w448 -> [w451] mode=indexing
                n163 = Unbundle(w451) -> (w450:dbl, w449:dbl)  [unwired: 1 out]
                n164 = Bundle(w450, w449) -> (w452:cluster{dbl, dbl})  [unwired: 1 out]
              }
            }
            frame False {
              n165 = call "CRYCurve Cut to Range.vi"("Axis type (Lin)"=0, "Range variable (x)"=enum16{"x", "y", "z"}."x" ("Range variable"), "Search range"=w457, "Curve in"=w458) -> ("Cut curve out"=w454:cluster{"x":dbl, "y":dbl, "z":dbl}[])  [unwired: 7 out]
              n166 = for {
                tunnel: w454 -> [w462] mode=indexing
                tunnel: [w459] -> w453 mode=indexing
                tunnel: [w459] -> _ mode=indexing
                n167 = Unbundle By Name(w462) -> ("x"=w461:dbl, "y"=w460:dbl)
                n168 = Bundle("x"=w461, "y"=w460) -> (w459:cluster{"x":dbl, "y":dbl})  [unwired: 1 out]
              }
            }
          }
        }
      }
      n169 = call "CRYCCITT_LR.vi"("Weight [Hz,dB]"=w425, "Freq. Response [Hz,dB]"=w437, "Exponent"=w429, "dB Correction [dB]"=0.0) -> ("LR [dB]"=w436:dbl)  [unwired: 1 out]
    }
    frame "ITU-T STMR" {
      w480 = u16 0  # dB
      w481 = 1.0  # dB ref (1Pa/Pa)
      (unwired) 0.225  # Exponent
      n170 = Unbundle By Name(w473) -> ("Y unit"=w474:string)
      n171 = call "CRYSpiltOnlyUnit.vi"("In Unit String"=w474) -> ("Out Unit String"=w472:string)  [unwired: 10 in]
      n172 = call "CRYUnits Conversion.vi"("Axis to change units"=enum16{"x", "y", "z"}."y", "New dB ref"=w481, "Custom unit in"=w472, "New data (dB/Lin)"=w480, "Data in"=w473) -> ("Data with new units"=w477:T1)  [unwired: 6 out]
      n173 = Unbundle By Name(w477) -> ("Curve"=w484:cluster{"x":dbl, "y":dbl, "z":dbl}[])
      n174 = for {
        tunnel: w484 -> [w512] mode=indexing
        tunnel: [w509] -> w483 mode=indexing
        n175 = Unbundle By Name(w512) -> ("x"=w511:dbl, "y"=w510:dbl)
        n176 = Bundle("x"=w511, "y"=w510) -> (w509:cluster{"x":dbl, "y":dbl})  [unwired: 1 out]
      }
      n177 = case shown="True" w471 {
        tunnel: [w487 w488] -> w469
        tunnel: w470 -> [w487 _]
        tunnel: w468 -> [_ w491]
        tunnel: w467 -> [_ w489]
        frame False {
        }
        frame True {
          n178 = call "CRYRead Weighting.vi"("Weighting filename"="ITU-T STMR Weighting.txt") -> ("Array"=w490:cluster{dbl, dbl, dbl}[])  [unwired: 9 in]
          n179 = case shown="True" w489 {
            tunnel: w491 -> [_ w504]
            tunnel: w490 -> [w494 w501]
            tunnel: [w493 w499] -> w488
            frame True {
              n180 = for {
                tunnel: [w498] -> w493 mode=indexing
                tunnel: [w495] -> _ mode=indexing
                tunnel: w494 -> [w495] mode=indexing
                n181 = Unbundle(w495) -> (w497:dbl, w496:dbl)  [unwired: 1 out]
                n182 = Bundle(w497, w496) -> (w498:cluster{dbl, dbl})  [unwired: 1 out]
              }
            }
            frame False {
              n183 = call "CRYCurve Cut to Range.vi"("Axis type (Lin)"=0, "Range variable (x)"=enum16{"x", "y", "z"}."x" ("Range variable"), "Search range"=w504, "Curve in"=w501) -> ("Cut curve out"=w500:cluster{"x":dbl, "y":dbl, "z":dbl}[])  [unwired: 7 out]
              n184 = for {
                tunnel: w500 -> [w508] mode=indexing
                tunnel: [w505] -> w499 mode=indexing
                tunnel: [w505] -> _ mode=indexing
                n185 = Unbundle By Name(w508) -> ("x"=w507:dbl, "y"=w506:dbl)
                n186 = Bundle("x"=w507, "y"=w506) -> (w505:cluster{"x":dbl, "y":dbl})  [unwired: 1 out]
              }
            }
          }
        }
      }
      n187 = call "CRYCCITT_LR.vi"("Weight [Hz,dB]"=w469, "Freq. Response [Hz,dB]"=w483, "Exponent"=w475, "dB Correction [dB]"=0.0) -> ("LR [dB]"=w482:dbl)  [unwired: 1 out]
    }
    frame "Attack Time", "Release Time" {
      n188 = Multiply(x=w540, y=0.01) -> (x*y=w517:dbl)
      n189 = Equal?(x="Attack Time" ("Operator 1"), y=w515) -> (x = y?=w514:bool)
      n190 = call "CRYAttack and Release.vi"("Sine waves"=w534, "Attack"=w533, "Search range"=w536, "% recovery"=w517, "All points"=w535, "Sampling rate"=w542, "Attack? (T)"=w514, "Data in"=w538) -> ("dy"=w513:dbl, "Attack or release time"=w518:dbl)  [unwired: 2 out]
      n191 = Search/Split String(string=w524, search string/char (-)="/" ("search char (-)")) -> (substring before match=w528:string, match + rest of string=w530:string, offset of match=w526:i32)  [unwired: 1 out]
      n192 = String Subset(string=w530, offset (0)=1) -> (substring=w531:string)  [unwired: 1 in]
      n193 = Greater Or Equal To 0?(x=w526) -> (x >= 0?=w527:bool)
      n194 = Select(t=w531, s=w527, f=w528) -> (s? t:f=w522:string)
      n195 = Format Into String(format string="dB re %.p %s", w519, w522) -> (resulting string=w521:string)  [unwired: 2 in, 1 out]
      n196 = Bundle By Name(cluster=w538, "Y data"=u16 0 ("Bundle Element"), "Y unit"=w521, "Y dB ref"=w519) -> (w537:T1)
    }
    frame "Zwicker Loudness" {
      n197 = call "CRYCalc zWicker Loudness.vi"("Zwicker_X-axis"=w551, "Zwicker_spectrum"=w550, "Data in"=w546) -> ("z"=w547:dbl, "y"=w548:dbl, "x"=w549:dbl, "Curve"=w545:cluster{"x":dbl, "y":dbl, "z":dbl}[])  [unwired: 5 in]
      n198 = Bundle By Name(cluster=w546, "Curve"=w545) -> (w544:T1)
    }
  }
  "value" <- w40
  "Frequency" <- w41
  "index" <- w52
  "Q" <- w39
  n199 = case shown="0, Default" "Zwicker_X-axis" {
    tunnel: ["Hz" ("X unit") "Bark" ("X unit")] -> w12
    frame 0, Default {
    }
    frame 1 {
    }
  }
  n200 = Equal?(x="Statistical Operator", y=u16 4) -> (x = y?=w34:bool)
  n201 = Equal?(x="Statistical Operator", y=u16 5) -> (x = y?=w33:bool)
  n202 = Not A Number/Path/Refnum?(number/path/refnum=w39) -> (NaN/Path/Refnum?=w43:bool)
  n203 = Or(x=w34, y=w33) -> (x .or. y?=w32:bool)
  n204 = Not A Number/Path/Refnum?(number/path/refnum=w41) -> (NaN/Path/Refnum?=w49:bool)
  n205 = case shown="False" w32 {
    tunnel: w43 -> [w558 _]
    tunnel: [w557 "Q" ("Z unit")] -> w42
    tunnel: w14 -> [w556 _]
    tunnel: "Statistical Operator" -> [w555 _]
    frame False {
      n206 = case shown="Default" w555 {
        tunnel: w558 -> [w563 _]
        tunnel: [w562 "Sone" ("Z unit")] -> w557
        tunnel: w556 -> [w560 _]
        frame Default {
          n207 = Unbundle By Name(w560) -> ("Z unit"=w559:string)
          n208 = Select(t="", s=w563, f=w559) -> (s? t:f=w562:string)
        }
        frame 15 {
        }
      }
    }
    frame True {
    }
  }
  n209 = Bundle By Name(cluster=w14, "X unit"=w12, "Y unit"="Phon") -> (→"Ranged data out(Curve)":T1)
  n210 = Bundle("x"=w41, "y"=w40, "z"=w39) -> (w38:cluster{"x":dbl, "y":dbl, "z":dbl})  [unwired: 1 in]
  n211 = Select(t="", s=w49, f=w24) -> (s? t:f=w48:string)
  n212 = Build Array(w38) -> (w37:cluster{"x":dbl, "y":dbl, "z":dbl}[])
  n213 = Bundle By Name(cluster=w14, "X unit"=w48, "single val"=TRUE, "Z unit"=w42, "Curve"=w37) -> (→"Ranged data out(Value)":T1)
